vi "PV HLT5xx background display active.vi"(7 "Adress of unit":u16=1 min=1 max=999 step=1, 8 "error in (no error)":errorcluster, 9 "set background display active":u16(ring) items=["background display deactivated", "background display activated"], 10 "Parameter\nread only<->describe":bool, 11 "VISA session":refnum<visa-resource-name>) -> (0 "error out":errorcluster, 1 "background display active out":u16(ring) items=["background display deactivated", "background display activated"], 2 "response (data)":string, 3 "dup VISA session":refnum<visa-resource-name>)   [LabVIEW 2021, in "Pfeiffer Vacuum.lvlib"]
doc: "This VI allows you to set or check the \"Dbackground display active (Para 644)\" on the SmartTest (HLT5xx)."
uses:
  <instrlib>/Pfeiffer Vacuum/Pfeiffer Vacuum.lvlib
panel:
  # "background display active"
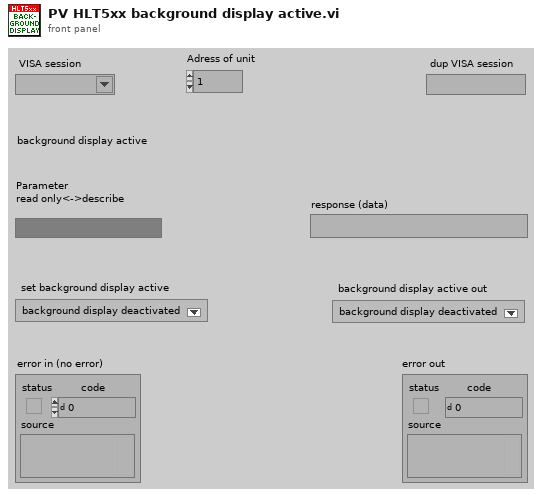
[diagram p1: front panel]
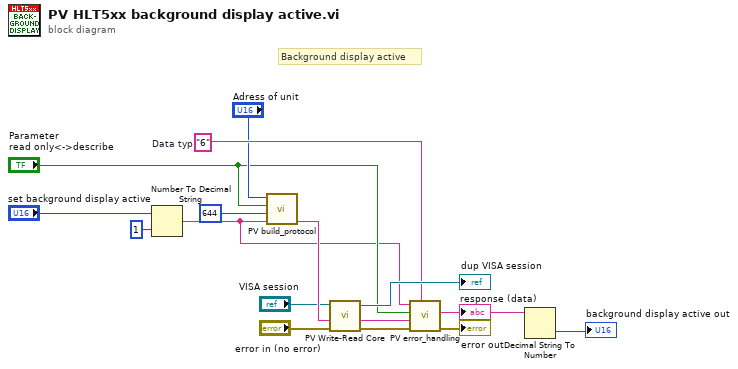
[diagram p0: block diagram]
diagram:
  w11 = "6"  # Data typ
  # "Background display active"
  n1 = Number To Decimal String(number="set background display active", width (-)=i16 1 ("Breite (-)")) -> (decimal integer string=w3:string)
  n2 = call <instrlib>:"PV build_protocol.vi"("Data"=w3, "Parameter-number"=u16 644, "parameter\nread<->describe"="Parameter\nread only<->describe", "Adress"="Adress of unit") -> ("output"=w15:string)  [unwired: 3 in]
  n3 = call <instrlib>:"PV Write-Read Core.vi"("error in"="error in (no error)", "Write data in"=w15, "VISA session"="VISA session") -> ("error out"=w13:errorcluster, "response (data) out"=w14:string, "dup VISA session"=→"dup VISA session":refnum<visa-resource-name>)  [unwired: 2 in]
  n4 = call <instrlib>:"PV error_handling.vi"("Data Typ in"=w11, "error in"=w13, "response (data) in"=w14, "Parameter\nread only<->describe"="Parameter\nread only<->describe", "data in"=w3) -> ("error out"=→"error out":errorcluster, "Data out"=w9:string)  [unwired: 4 in, 1 out]
  "response (data)" <- w9
  n5 = Decimal String To Number(string=w9) -> (number=→"background display active out":i32)  [unwired: 2 in, 1 out]
